vi "Validate Command.vi"(4 "error in (no error)":errorcluster, 7 "Serial in":refnum<visa-resource-name>) -> (0 "error out":errorcluster, 2 "Valid?":bool, 3 "Serial Out":refnum<visa-resource-name>)   [LabVIEW 2019]
uses:
  <vilib>/Utility/error.llb/Error Cluster From Error Code.vi
  <vilib>/ErrorRing/Error Ring.xnode
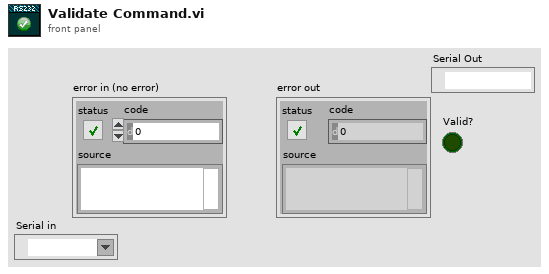
[diagram p1: front panel]
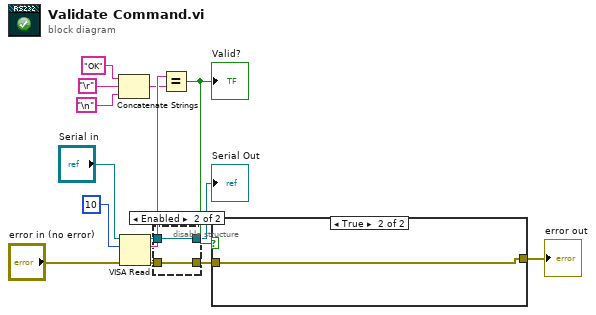
[diagram p0: block diagram]
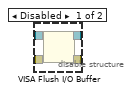
[diagram p2: hidden frame]
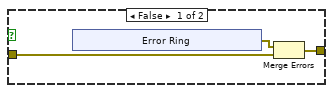
[diagram p3: hidden frame]
diagram:
  n1 = Concatenate Strings("OK" ("y"), "\r", "\n") -> (w3:string)
  n2 = VISA Read(VISA resource name="Serial in", byte count=u32 10, error in (no error)="error in (no error)") -> (VISA resource name out=w8:refnum<visa-resource-name>, read buffer=w4:string, error out=w6:errorcluster)  [unwired: 1 out]
  n3 = disable-structure shown="Enabled" {
    disable-tunnel: w8 -> [w18 w20]
    disable-tunnel: [w17 w20] -> w7
    disable-tunnel: w6 -> [w16 w19]
    disable-tunnel: [w15 w19] -> w5
    frame Disabled {
      n4 = VISA Flush I/O Buffer(VISA resource name=w18, error in (no error)=w16) -> (VISA resource name out=w17:refnum<visa-resource-name>, error out=w15:errorcluster)  [unwired: 1 in]
    }
    frame Enabled {
    }
  }
  "Serial Out" <- w7
  n5 = Equal?(x=w4, y=w3) -> (x = y?=w9:bool)
  "Valid?" <- w9
  n6 = case shown="True" w9 {
    tunnel: [w23 w29] -> w10
    tunnel: w5 -> [w21 w29]
    frame False {
      n7 = xnode "Error Ring"() -> ("error out"=w22:errorcluster)
      n8 = Merge Errors(w22, w21) -> (w23:errorcluster)
    }
    frame True {
    }
  }
  "error out" <- w10
